vi "Duplicate Routing Channel RTM.vi"(8 "error in (no error)":errorcluster, 11 "Node Ptr":u64 format="%.0x") -> (0 "error out":errorcluster)   [LabVIEW 2020, in "Routing and Faulting System Explorer.lvlib"]
uses:
  Routing and Faulting System Explorer.lvlib
  9b785d74-dca3-4762-b15d-51e0b6148e04.vi
  Scripting/Routing and Faulting Scripting.lvlib
  <vilib>/NI VeriStand/Custom Device Tools/Custom Device Utility Library/Custom Device Utility Library.lvlib
  <vilib>/NI VeriStand/Custom Device API/Custom Device API.lvlib
panel:
  in  "Tag":string
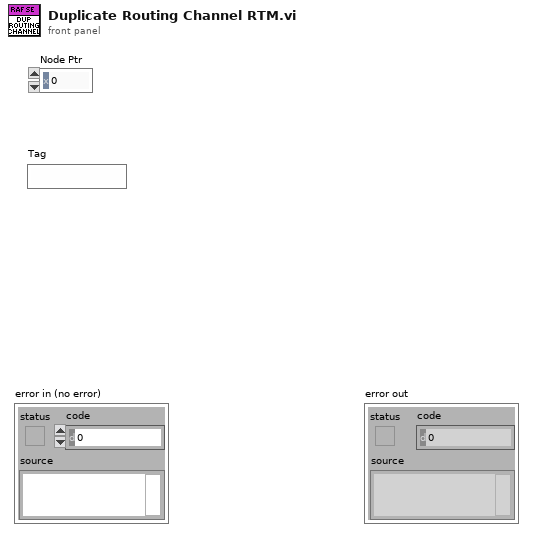
[diagram p1: front panel]
types:
  T1 = typedef "Routing and Faulting Shared.lvlib/Channel States.ctl" = T2[]
  T2 = typedef "Routing and Faulting Shared.lvlib/Routing State.ctl" = cluster{"Name":string, "Description":string, "Value":i32, "Connection List":T3[]}
  T3 = typedef "Routing and Faulting Shared.lvlib/Connection.ctl" = cluster{"Module":string, "Source":string, "Destination":string}
  T4 = typedef "Custom Device API.lvlib/Custom Device Item Ref.ctl" = u64
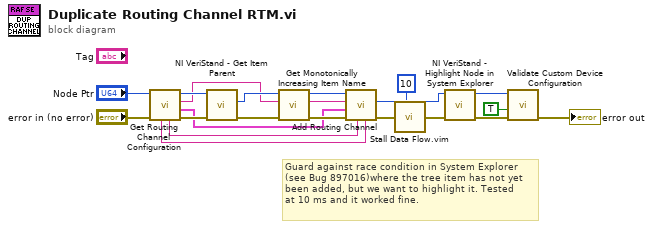
[diagram p0: block diagram]
diagram:
  # "Guard against race condition in System Explorer\n(see Bug 897016)where the tree item has not yet\nbeen added, but we want to highlight it. Tested\nat 10 ms and it worked fine."
  n1 = call "Get Routing Channel Configuration.vi"("error in"="error in (no error)", "routing channel in"="Node Ptr") -> ("error out"=w14:errorcluster, "state configurations"=w9:T1, "routing channel name"=w11:string, "routing channel out"=w13:T4, "initial state"=w8:string, "description"=w7:string)  [unwired: 4 in]
  n2 = call <vilib>:"NI VeriStand - Get Item Parent.vi"("error in (no error)"=w14, "Item Ref in"=w13) -> ("error out"=w10:errorcluster, "Parent Ref"=w12:T4)  [unwired: 6 in, 2 out]
  n3 = call "Get Monotonically Increasing Item Name.vi"("error in (no error)"=w10, "Desired Name"=w11, "Section Ptr"=w12) -> ("error out"=w20:errorcluster, "New Item Name"=w19:string, "Section Ptr out"=w21:T4)  [unwired: 6 in]
  n4 = call "Add Routing Channel.vi"("description"=w7, "initial state"=w8, "error in"=w20, "state configurations"=w9, "channel name"=w19, "routing channels in"=w21) -> ("error out"=w18:errorcluster, "routing channel"=w17:T4)  [unwired: 3 in, 1 out]
  n5 = call "Stall Data Flow.vim"("value in"=w18, "milliseconds to wait"=u32 10) -> ("value out"=w6:errorcluster)  [unwired: 1 out]
  n6 = call <vilib>:"NI VeriStand - Highlight Node in System Explorer.vi"("error in (no error)"=w6, "Item Ref in"=w17) -> ("error out"=w4:errorcluster, "Node Ptr dup"=w3:T4)  [unwired: 8 in]
  n7 = call "Validate Custom Device Configuration.vi"("error in (no error)"=w4, "Force Validation (F)"=TRUE, "Routing and Faulting Custom Device Ref"=w3) -> ("error out"=→"error out":errorcluster)  [unwired: 6 in, 2 out]
